vi "Tag Write.vi"(8 "error in (no error)":errorcluster, 11 "Tag IN":T1={"Tag Name"=["LStatus", "RStatus", "LTargetTemp", "LTemp1", "LTemp2", "LTemp3", "LTemp4", "LTemp5", "LTemp6", "RTargetT", "RTemp1", "RTemp2", "RTemp3", "RTemp4", "RTemp5", "RTemp6", "LWO", "LOPID", "LDate", "LTime", "LModel", "LAgingTime", "LAgingTemp", "LStartTime", "LEndTime", "RWO", "ROPID", "RDate", "RTime", "RModel", "RAgingTime", "RAgingTemp", "RStartTime", "REndTime"], "Tag Type"=[enum."String", enum."String", enum."Double", enum."Double", enum."Double", enum."Double", enum."Double", enum."Double", enum."Double", enum."Double", enum."Double", enum."Double", enum."Double", enum."Double", enum."Double", enum."Double", enum."String", enum."String", enum."String", enum."String", enum."String", enum."String", enum."String", enum."String", enum."String", enum."String", enum."String", enum."String", enum."String", enum."String", enum."String", enum."String", enum."String", enum."String"], "Tag Data"=[], "Skyline Array"=[]}) -> (0 "error out":errorcluster)   [LabVIEW 2017]
uses:
  Tag.ctl
  <vilib>/Skyline/Tag/Shared/typedefs/DataType.ctl
  <vilib>/Skyline/Tag/Wrapper/Wrapper_class/NI Skyline Tag.lvclass
  <vilib>/Skyline/Tag/Wrapper/Wrapper_class/Generate Tag Cluster (DBL) 2.vi
  <vilib>/Skyline/Tag/Wrapper/Wrapper_class/Generate Tag Cluster (I32) 2.vi
  <vilib>/Skyline/Tag/Wrapper/Wrapper_class/Generate Tag Cluster (String) 2.vi
  <vilib>/Skyline/Tag/Wrapper/Wrapper_class/Generate Tag Cluster (Boolean) 2.vi
  <vilib>/Skyline/Tag/Wrapper/Wrapper_class/Generate Tag Cluster (U64) 2.vi
  <vilib>/Skyline/Tag/Wrapper/Wrapper_class/Generate Tag Cluster (Timestamp) 2.vi
  <vilib>/Skyline/Tag/Shared/NI Skyline Tag.lvlib
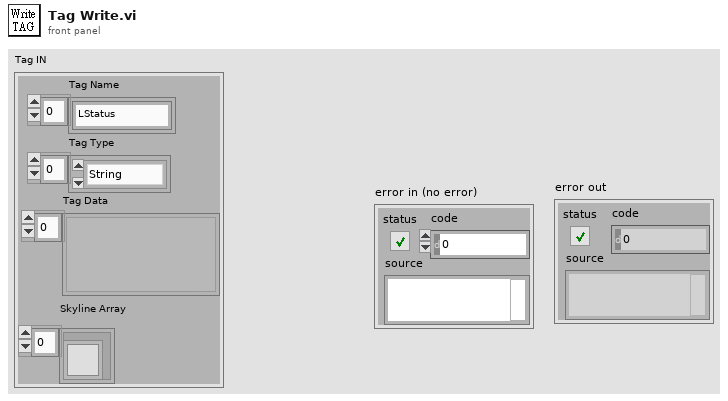
[diagram p1: front panel]
types:
  T1 = typedef "Tag.ctl" = cluster{"Tag Name":string[], "Tag Type":T2[], "Tag Data":variant[], "Skyline Array":refnum<class "NI Skyline Tag.lvclass">[]}
  T2 = typedef "NI Skyline Tag.lvlib/DataType.ctl" = enum32{"Double", "I32", "String", "Boolean", "U64", "Timestamp"}
  T3 = typedef "NI Skyline Tag.lvclass/Tag Value Cluster Wrapper.ctl" = cluster{"Configuration":refnum<class "NI Skyline Configuration.lvclass">, "Tag Cluster":T4}
  T4 = typedef "NI Skyline Tag.lvlib/Tag Value Cluster.ctl" = cluster{"Path":string, "Data Type":T2, "Value":string, "Time Stamp":timestamp}
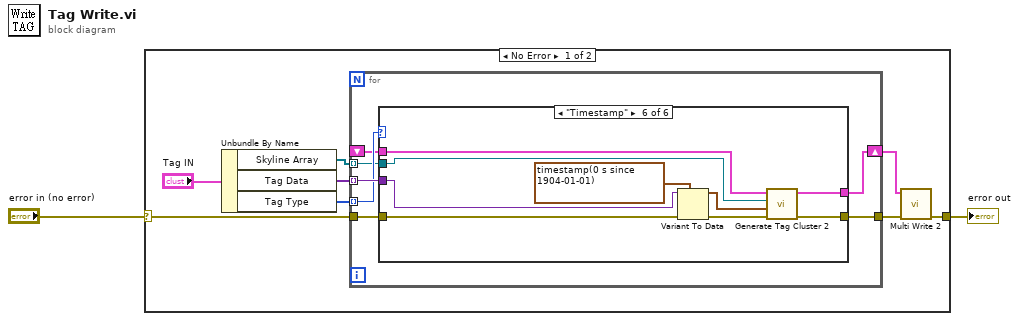
[diagram p0: block diagram]
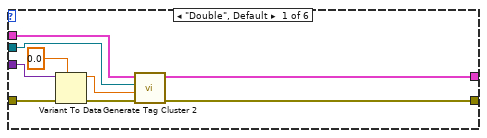
[diagram p2: hidden frame]
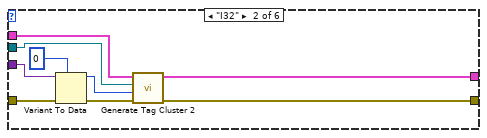
[diagram p3: hidden frame]
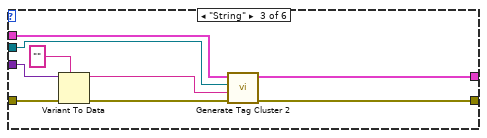
[diagram p4: hidden frame]
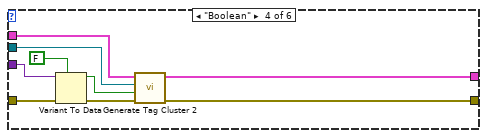
[diagram p5: hidden frame]
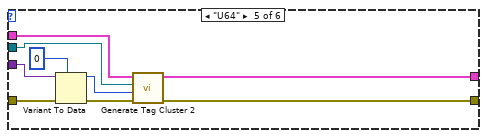
[diagram p6: hidden frame]
diagram:
  n1 = case shown="No Error" "error in (no error)" {
    selector: "error in (no error)" -> [w5 w72]
    tunnel: [w3 w72] -> w1
    frame No Error {
      n2 = Unbundle By Name("Tag IN") -> ("Skyline Array"=w9:refnum<class "NI Skyline Tag.lvclass">[], "Tag Data"=w8:variant[], "Tag Type"=w7:T2[])
      n3 = for {
        tunnel: w9 -> [w15] mode=indexing
        tunnel: w8 -> [w17] mode=indexing
        tunnel: w7 -> [w16] mode=indexing
        shift-right: [w14] -> w6
        shift-left: _ -> [w13]
        tunnel: w5 -> [w12]
        tunnel: [w11] -> w4
        n4 = case shown="\"Timestamp\"" w16 {
          tunnel: w17 -> [w25 w35 w44 w53 w62 w71]
          tunnel: w15 -> [w26 w33 w43 w52 w61 w70]
          tunnel: [w24 w32 w42 w51 w60 w69] -> w14
          tunnel: [w23 w31 w41 w50 w59 w68] -> w11
          tunnel: w13 -> [w20 w29 w38 w47 w56 w65]
          tunnel: w12 -> [w19 w28 w36 w45 w54 w63]
          frame "Double", Default {
            n5 = Variant To Data(error in=w19, type=0.0 ("value"), Variant=w25) -> (data=w21:dbl, error out=w18:errorcluster)
            n6 = call-poly <vilib>:"Generate Tag Cluster 2.vi"("error in (no error)"=w18, "value"=w21, "tag in"=w26, "tag clusters in"=w20) -> ("error out"=w23:errorcluster, "tag clusters out"=w24:T3[])  [unwired: 5 in, 1 out]
          }
          frame "I32" {
            n7 = Variant To Data(error in=w28, type=0, Variant=w35) -> (data=w30:i32, error out=w27:errorcluster)
            n8 = call-poly <vilib>:"Generate Tag Cluster 2.vi"("error in (no error)"=w27, "value"=w30, "tag in"=w33, "tag clusters in"=w29) -> ("error out"=w31:errorcluster, "tag clusters out"=w32:T3[])  [unwired: 5 in, 1 out]
          }
          frame "String" {
            n9 = Variant To Data(error in=w36, type="", Variant=w44) -> (data=w39:string, error out=w37:errorcluster)
            n10 = call-poly <vilib>:"Generate Tag Cluster 2.vi"("error in (no error)"=w37, "value"=w39, "tag in"=w43, "tag clusters in"=w38) -> ("error out"=w41:errorcluster, "tag clusters out"=w42:T3[])  [unwired: 5 in, 1 out]
          }
          frame "Boolean" {
            n11 = Variant To Data(error in=w45, type=FALSE, Variant=w53) -> (data=w48:bool, error out=w46:errorcluster)
            n12 = call-poly <vilib>:"Generate Tag Cluster 2.vi"("error in (no error)"=w46, "value"=w48, "tag in"=w52, "tag clusters in"=w47) -> ("error out"=w50:errorcluster, "tag clusters out"=w51:T3[])  [unwired: 5 in, 1 out]
          }
          frame "U64" {
            n13 = Variant To Data(error in=w54, type=u64 0, Variant=w62) -> (data=w57:u64, error out=w55:errorcluster)
            n14 = call-poly <vilib>:"Generate Tag Cluster 2.vi"("error in (no error)"=w55, "value"=w57, "tag in"=w61, "tag clusters in"=w56) -> ("error out"=w59:errorcluster, "tag clusters out"=w60:T3[])  [unwired: 5 in, 1 out]
          }
          frame "Timestamp" {
            n15 = Variant To Data(error in=w63, type=timestamp(0 s since 1904-01-01), Variant=w71) -> (data=w66:timestamp, error out=w64:errorcluster)
            n16 = call-poly <vilib>:"Generate Tag Cluster 2.vi"("error in (no error)"=w64, "value"=w66, "tag in"=w70, "tag clusters in"=w65) -> ("error out"=w68:errorcluster, "tag clusters out"=w69:T3[])  [unwired: 5 in, 1 out]
          }
        }
      }
      n17 = call <vilib>:"Multi Write 2.vi"("error in (no error)"=w4, "tag clusters"=w6) -> ("error out"=w3:errorcluster)  [unwired: 9 in]
    }
    frame Error {
    }
  }
  "error out" <- w1
